vi "WLAN_Descrambler.vi"(0 "scrambler initial bits":i8[](array[numeric]), 1 "data bits":i8[](array[numeric])) -> (6 "scrambled bits":i8[](array[numeric]))   [LabVIEW 2022 SP3]
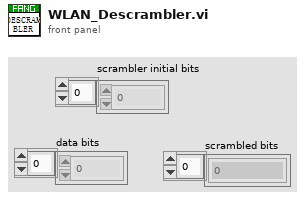
[diagram p1: front panel]
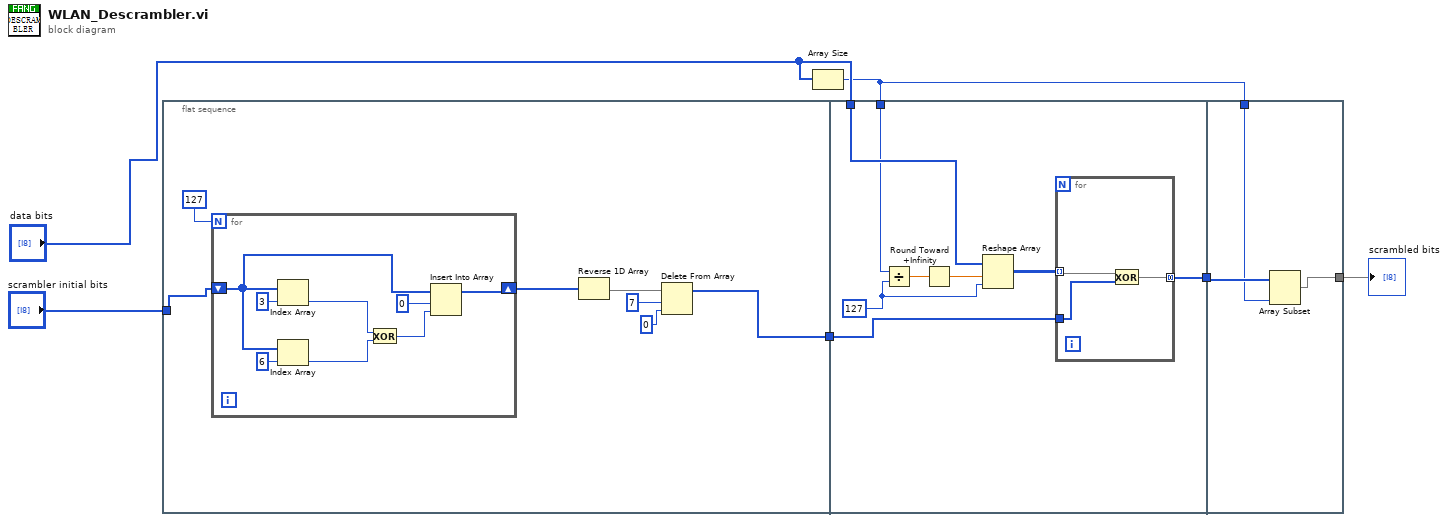
[diagram p0: block diagram]
diagram:
  n1 = flat-sequence {
    tunnel: [w8] -> w6
    tunnel: "scrambler initial bits" -> [w7]
    tunnel: w6 -> [w25]
    tunnel: "data bits" -> [w23]
    tunnel: [w24] -> w3
    tunnel: w1 -> [w22]
    tunnel: [w33] -> w5
    tunnel: w3 -> [w35]
    tunnel: w1 -> [w34]
    frame #0 {
      n2 = for {
        N: 127 -> [_]
        shift-right: [w14] -> w9
        shift-left: w7 -> [w17]
        n3 = Index Array(array=w17, index=3) -> (element=w19:i8)
        n4 = Index Array(array=w17, index=6) -> (element=w18:i8)
        n5 = Exclusive Or(1:w18, 2:w19) -> (0:w15:i8)
        n6 = Insert Into Array(array=w17, index=0, new element=w15) -> (w14:i8[])
      }
      n7 = Reverse 1D Array(array=w9) -> (reversed array=w10:i8[])
      n8 = Delete From Array(array=w10, length=7, index=0) -> (array with subset deleted=w8:i8[])  [unwired: 1 out]
    }
    frame #1 {
      w27 = 127
      n9 = Divide(x=w22, y=w27) -> (x/y=w29:dbl)
      n10 = Round Toward +Infinity(x=w29) -> (ceil(x): smallest int >= x=w28:dbl)
      n11 = Reshape Array(w23, w28, w27) -> (w26:i8[][])
      n12 = for {
        tunnel: w26 -> [w30] mode=indexing
        tunnel: w25 -> [w32]
        tunnel: [w31] -> w24 mode=concatenating
        n13 = Exclusive Or(1:w32, 2:w30) -> (0:w31:i8[])
      }
    }
    frame #2 {
      n14 = Array Subset(array=w35, length=w34) -> (w33:i8[])  [unwired: 1 in]
    }
  }
  n15 = Array Size(array="data bits") -> (size(s)=w1:i32)
  "scrambled bits" <- w5
